vi "set_resolution.vi"(8 "error in (no error)":errorcluster, 9 "y resolution":i32, 10 "x resolution":i32, 11 "FPGAWrapperMH120124FrameScan_PXI7813R in":refnum<class "FPGAWrapperMH120124FrameScan_PXI7813R.lvclass">) -> (0 "error out":errorcluster, 3 "FPGAWrapperMH120124FrameScan_PXI7813R out":refnum<class "FPGAWrapperMH120124FrameScan_PXI7813R.lvclass">)   [LabVIEW 2010, in "FPGAWrapperMH120124FrameScan_PXI7813R.lvclass"]
uses:
  FPGAWrapperMH120124FrameScan_PXI7813R.lvclass
  FPGAWrapperMH120124FrameScan_PXI7813R.lvclass/FPGAWrapperMH120124FrameScan_PXI7813R.ctl
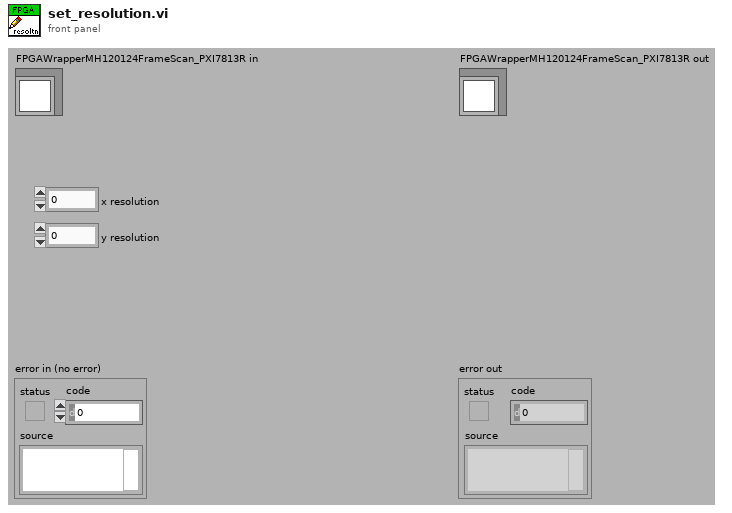
[diagram p1: front panel]
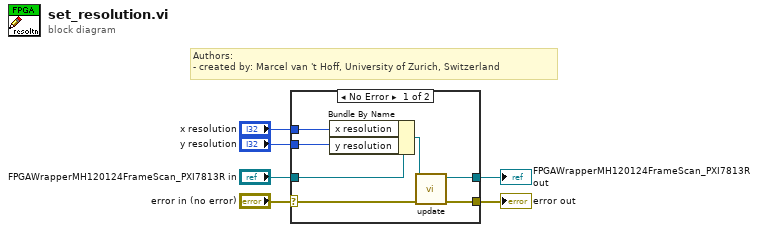
[diagram p0: block diagram]
diagram:
  # "Authors: \n- created by: Marcel van 't Hoff, University of Zurich, Switzerland"
  n1 = case shown="No Error" "error in (no error)" {
    selector: "error in (no error)" -> [w8 w14]
    tunnel: [w7 w14] -> w5
    tunnel: [w9 w15] -> w3
    tunnel: "FPGAWrapperMH120124FrameScan_PXI7813R in" -> [w13 w15]
    tunnel: "y resolution" -> [w12 _]
    tunnel: "x resolution" -> [w11 _]
    frame No Error {
      n2 = Bundle By Name(cluster=w13, "x resolution"=w11, "y resolution"=w12) -> (w10:refnum<class "FPGAWrapperMH120124FrameScan_PXI7813R.lvclass">)
      n3 = call-dynamic "update.vi"("error in (no error)"=w8, "FPGAWrapperMH120124FrameScan_PXI7813R in"=w10) -> ("error out"=w7:errorcluster, "FPGAWrapperMH120124FrameScan_PXI7813R out"=w9:refnum<class "FPGAWrapperMH120124FrameScan_PXI7813R.lvclass">)  [unwired: 8 in]
    }
    frame Error {
    }
  }
  "error out" <- w5
  "FPGAWrapperMH120124FrameScan_PXI7813R out" <- w3
